vi "View.vi"(8 "error in (no error)":errorcluster, 10 "Context":refnum<class "Debug Process.lvclass">, 11 "Debug View in":refnum<class "Debug View.lvclass">) -> (0 "error out":errorcluster, 3 "Debug View out":refnum<class "Debug View.lvclass">)   [LabVIEW 2020, in "Debug View.lvclass"]
uses:
  Debug View.lvclass
  Process/Debug Process.lvclass
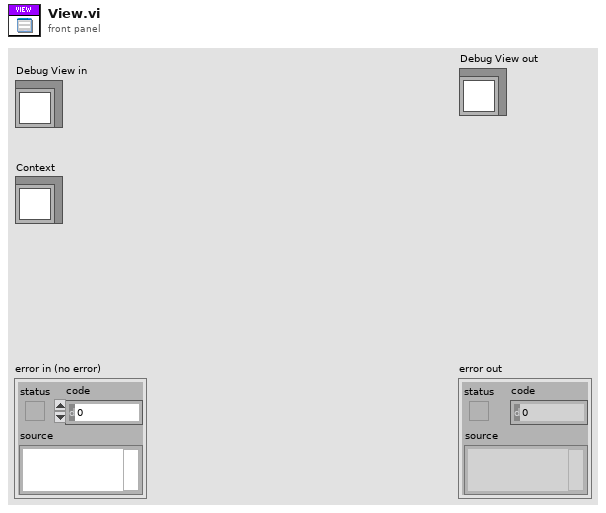
[diagram p1: front panel]
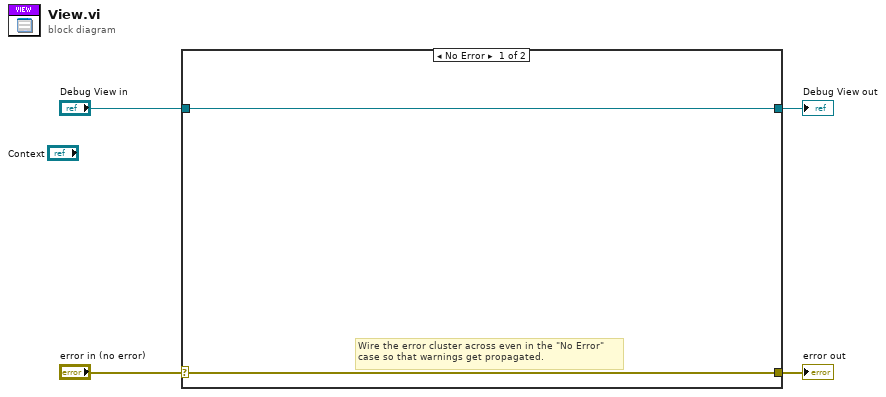
[diagram p0: block diagram]
diagram:
  n1 = case shown="No Error" "error in (no error)" {
    selector: "error in (no error)" -> [w5 w8]
    tunnel: [w5 w8] -> w3
    tunnel: [w6 w7] -> w1
    tunnel: "Debug View in" -> [w6 w7]
    frame No Error {
      # "Wire the error cluster across even in the \"No Error\"\ncase so that warnings get propagated."
    }
    frame Error {
    }
  }
  "error out" <- w3
  "Debug View out" <- w1
